vi "UnloadGraphVI_LS1.vi"(8 "ErrorIn(No Error)":errorcluster caption="entrée d'erreur (pas d'erreur)", 10 "GraphRef":refnum<vi>) -> (0 "sortie d'erreur":errorcluster)   [LabVIEW 2010]
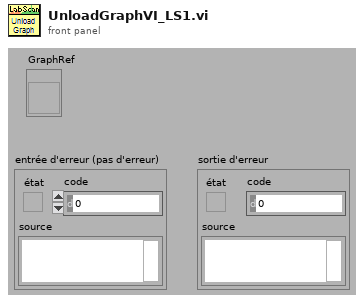
[diagram p1: front panel]
types:
  T1 = enum32{"Invalid", "Standard", "Closed", "Hidden", "Minimized", "Maximized"}
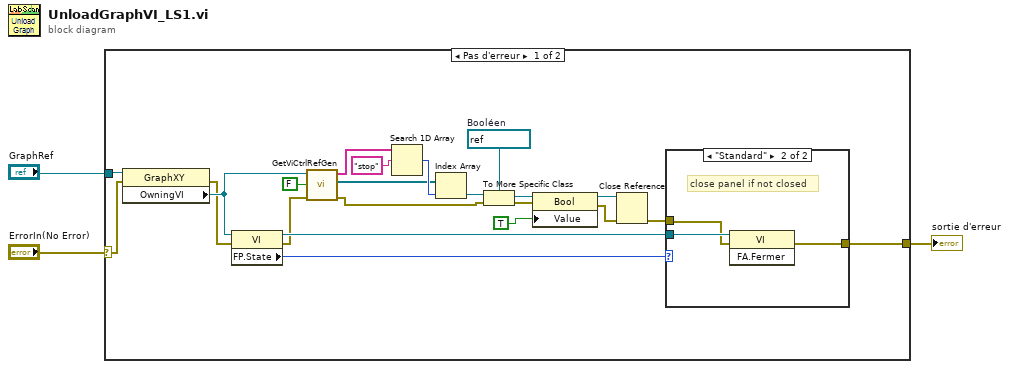
[diagram p0: block diagram]
diagram:
  n1 = case shown="Pas d'erreur" "ErrorIn(No Error)" {
    selector: "ErrorIn(No Error)" -> [w11 w30]
    tunnel: "GraphRef" -> [w12 _]
    tunnel: [w4 w30] -> w1
    frame No Error {
      w20 = refnum<vi> refnum  # Booléen
      n2 = property class="GraphXY"(reference=w12, error in=w11) -> (error out=w6:errorcluster, "OwningVI"=w7:refnum<vi>)  [unwired: 1 out]
      n3 = property class="VI"(reference=w7, error in=w6) -> (reference out=w8:refnum<vi>, error out=w5:errorcluster, "FP.State"=w10:T1)
      n4 = call <userlib>:"GetViCtrlRefGen.vi"("ErrorIn(No Error)"=w5, "InclTabCTrl"=FALSE, "VIRef"=w7) -> ("sortie d'erreur"=w17:errorcluster, "ControlsRefs"=w21:refnum<vi>[], "ControlsNames"=w24:string[])  [unwired: 6 in]
      n5 = Search 1D Array(1D array=w24, element="stop" ("élément")) -> (index of element=w22:i32)  [unwired: 1 in]
      n6 = Index Array(array=w21, index=w22) -> (element=w19:refnum<vi>)
      n7 = To More Specific Class(target class=w20, reference=w19, error in=w17) -> (specific class reference=w18:refnum<vi>, error out=w16:errorcluster)
      n8 = property class="Bool"(reference=w18, error in=w16, "Value"=TRUE) -> (reference out=w14:refnum<vi>, error out=w13:errorcluster)
      n9 = Close Reference(reference=w14, error in (no error)=w13) -> (error out=w9:errorcluster)
      n10 = case shown="\"Standard\"" w10 {
        tunnel: w9 -> [w26 w28]
        tunnel: [w26 w27] -> w4
        tunnel: w8 -> [_ w29]
        frame "Invalid", Default {
        }
        frame "Standard" {
          # "close panel if not closed"
          n11 = invoke class="VI" method="FA.Fermer"(reference=w29, error in=w28) -> (error out=w27:errorcluster)  [unwired: 1 in, 2 out]
        }
      }
    }
    frame Error {
    }
  }
  "sortie d'erreur" <- w1
